vi "ReadTextplain.vi"(8 "error in (no error)":errorcluster, 11 "object in":refnum<class "display_data Message.lvclass">) -> (0 "error out":errorcluster, 2 "text/plain":string, 3 "object out":refnum<class "display_data Message.lvclass">)   [LabVIEW 2018, in "ClientMessaging.lvlib" / "display_data Message.lvclass"]
uses:
  display_data Message.lvclass
  display_data Message.lvclass/display_data Message.ctl
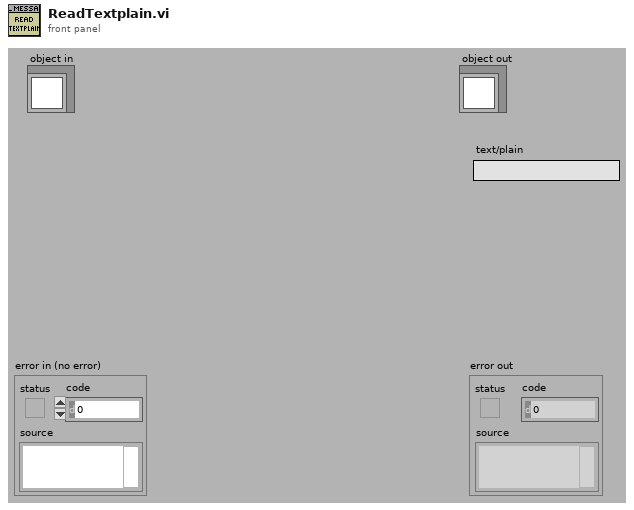
[diagram p1: front panel]
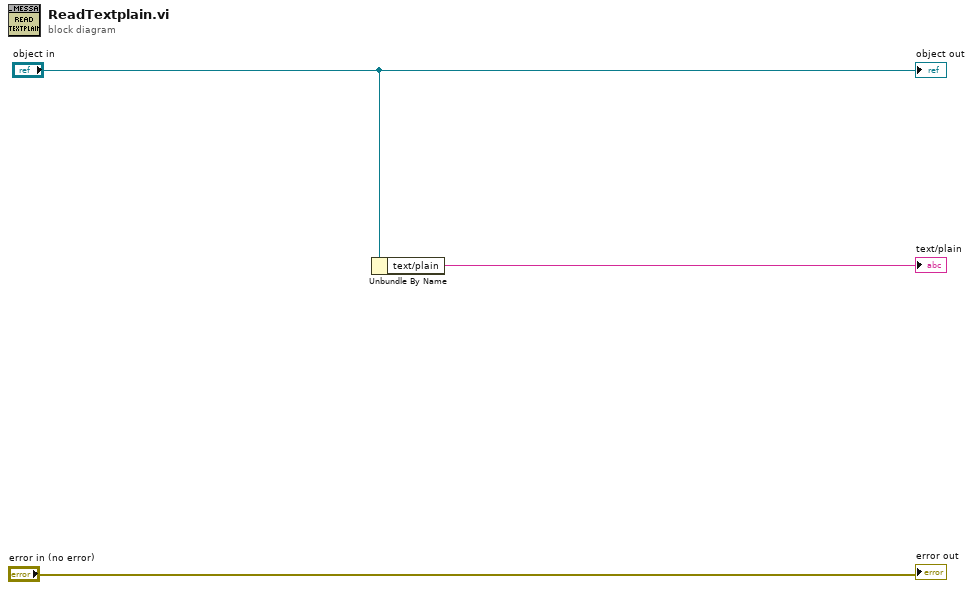
[diagram p0: block diagram]
diagram:
  n1 = Unbundle By Name("object in") -> ("text/plain"=→"text/plain":string)
  "error out" <- "error in (no error)"
  "object out" <- "object in"
